vi "XY Graph Plot ASCII File Format Dialog.vi"(8 "error in (no error)":errorcluster) -> (0 "error out":errorcluster, 1 "Number of Lines to Skip":i32, 2 "Column Header Line?":bool, 3 "Separator":string, 4 "OK":bool)   [LabVIEW 2019, in "XY Graph Add-Ons.lvlib"]
doc: "Displays a standard dialog box that prompts users to enter information, such as a user name and password.\n--------------------\n\nThis Express VI is configured as follows:\n\nMessage to Display to the User:Define File Format\nThe inputs are: \nNumber: Number of Lines to Skip:\nCheckbox: Header Line?\nText Entry Box: Separator:"
uses:
  XY Graph Add-Ons.lvlib
panel:
  in  "Separator:":string(combo)="Tab"
  in  "Column Header Line?":bool caption="Header Line?"
  in  "Number of Lines to Skip:":i32
  out "String":string="Define File Format:"
  in  "Cancel":bool
  in  "OK2":bool
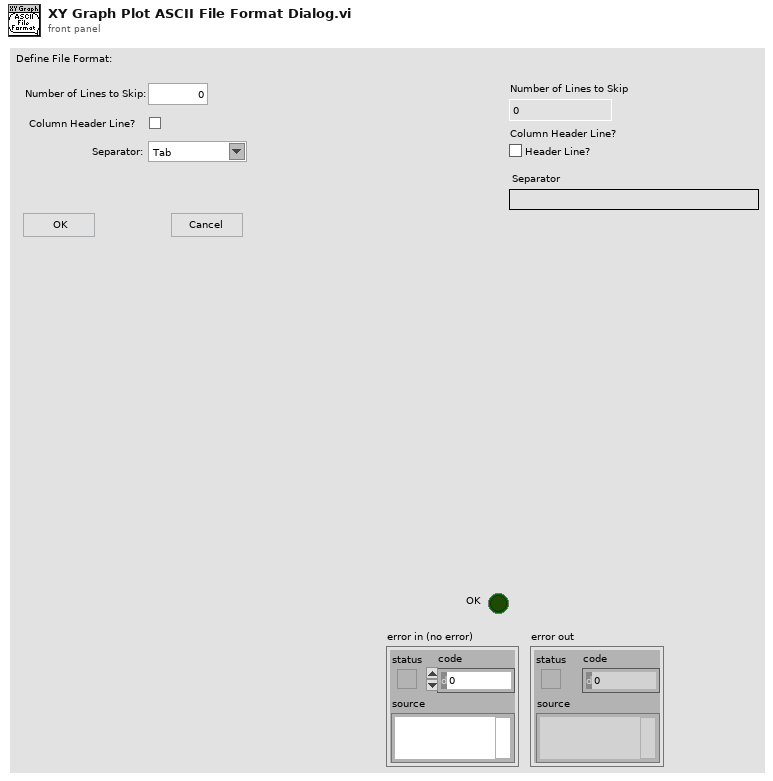
[diagram p1: front panel]
types:
  T1 = cluster{"Input Name":string, "Input Data Type":i32}[]
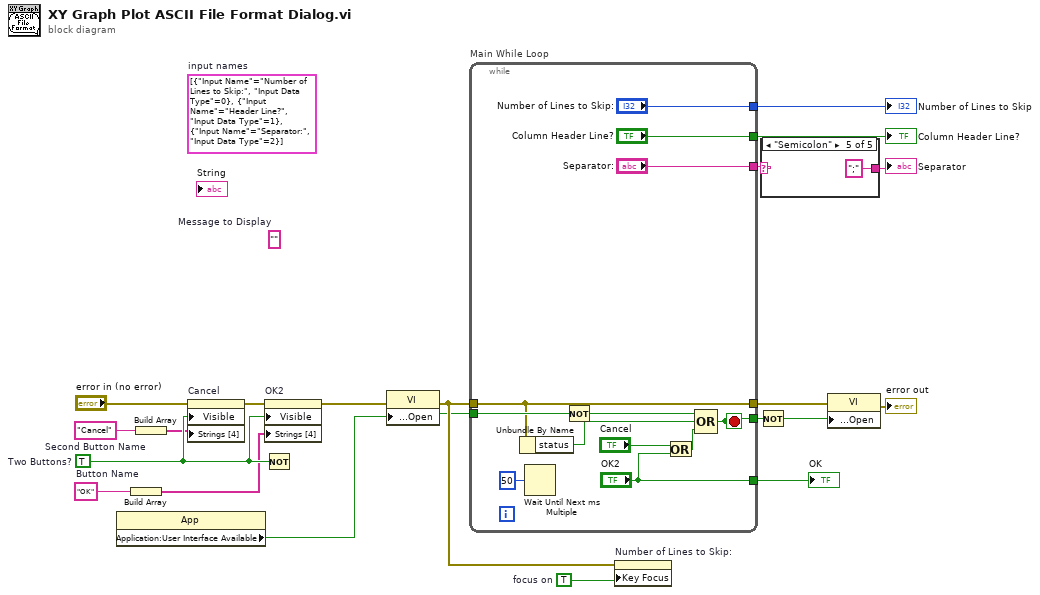
[diagram p0: block diagram]
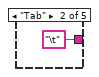
[diagram p3: hidden frame]
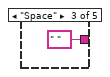
[diagram p4: hidden frame]
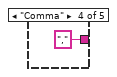
[diagram p5: hidden frame]
diagram:
  w6 = TRUE  # focus on
  (unwired) T1 [{"Input Name"="Number of Lines to Skip:", "Input Data Type"=0}, {"Input Name"="Header Line?", "Input Data Type"=1}, {"Input Name"="Separator:", "Input Data Type"=2}]  # input names
  w14 = "Cancel"  # Second Button Name
  w12 = "OK"  # Button Name
  (unwired) ""  # Message to Display
  w20 = TRUE  # Two Buttons?
  n1 = property class="App"() -> ("Application:User Interface Available"=w1:bool)  [unwired: 2 in, 2 out]
  n2 = Build Array(w12) -> (w13:string[])
  n3 = Build Array(w14) -> (w15:string[])
  n4 = property on="Cancel" class="Bool"(error in="error in (no error)", "Visible"=w20, "Strings [4]"=w15) -> (error out=w18:errorcluster)  [unwired: 1 in, 1 out]
  n5 = Not(x=w20) -> ()  [unwired: 1 out]
  n6 = property on="OK2" class="Bool"(error in=w18, "Visible"=w20, "Strings [4]"=w13) -> (error out=w4:errorcluster)  [unwired: 1 in, 1 out]
  n7 = property class="VI"(error in=w4, "Front Panel Window:Open"=w1) -> (error out=w11:errorcluster)  [unwired: 1 in, 1 out]
  n8 = while "Main While Loop" {
    tunnel: ["OK2"] -> w19
    tunnel: w1 -> [w29]
    tunnel: [w27] -> w16
    tunnel: w11 -> [w26]
    tunnel: [w26] -> w9
    tunnel: ["Number of Lines to Skip:"] -> w7
    tunnel: ["Column Header Line?"] -> w5
    tunnel: ["Separator:"] -> w3
    stop <- w27 stop-if-true
    n9 = Unbundle By Name(w26) -> ("status"=w24:bool)
    n10 = Wait Until Next ms Multiple(millisecond multiple=u32 50) -> ()  [unwired: 1 out]
    n11 = Not(x=w29) -> (.not. x?=w28:bool)
    n12 = Or(x="Cancel", y="OK2") -> (x .or. y?=w25:bool)
    n13 = Compound Arithmetic op=OR(w28, w24, w25) -> (w27:bool)
  }
  "OK" <- w19
  "Number of Lines to Skip" <- w7
  "Column Header Line?" <- w5
  n14 = property on="Number of Lines to Skip:" class="DigNum (strict)"(error in=w11, "Key Focus"=w6) -> ()  [unwired: 1 in, 2 out]
  n15 = Not(x=w16) -> (.not. x?=w17:bool)
  n16 = case shown="\"Semicolon\"" w3 {
    selector: w3 -> [w33 _ _ _ _]
    tunnel: [w33 "\t" " " "," ";"] -> w2
    frame "", Default {
    }
    frame "Tab" {
    }
    frame "Space" {
    }
    frame "Comma" {
    }
    frame "Semicolon" {
    }
  }
  "Separator" <- w2
  n17 = property class="VI"(error in=w9, "Front Panel Window:Open"=w17) -> (error out=→"error out":errorcluster)  [unwired: 1 in, 1 out]
